vi "VI01.vi"(9 "VC":dbl, 11 "VE's":dbl[](array[numeric])) -> (3 "VF":dbl)   [LabVIEW 2017]
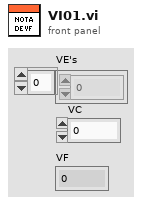
[diagram p1: front panel]
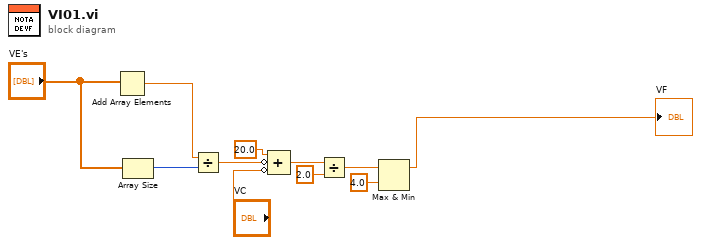
[diagram p0: block diagram]
diagram:
  n1 = Add Array Elements(numeric array="VE's") -> (sum=w3:dbl)
  n2 = Array Size(array="VE's") -> (size(s)=w2:i32)
  n3 = Divide(x=w3, y=w2) -> (x/y=w10:dbl)
  n4 = Compound Arithmetic op=ADD(20.0 ("value"), invert w10, invert "VC") -> (w9:dbl)
  n5 = Divide(x=w9, y=2.0 ("value")) -> (x/y=w8:dbl)
  n6 = Max & Min(x=w8, y=4.0) -> (max(x,y)=→"VF":dbl)  [unwired: 1 out]
